vi "Stop Core.vi"(10 "final error code":i32, 11 "Thermocouples in":refnum<class "Thermocouples.lvclass">=refnum) -> (3 "Thermocouples out":refnum<class "Thermocouples.lvclass">)   [LabVIEW 2015]
doc: "(<B>Filename</B>: Actor Framework.lvlib:Actor.lvclass:Stop Core.vi)\n\nDefines what the actor does before it stops. Use the <B>final error code</B> input to determine whether the actor shut down in response to an error.\n\nBy default, this method does nothing. A descendant class may override it to define behavior, such as shutting down any processes the actor initiated in its override of the Actor Core method."
uses:
  Thermocouples.lvclass
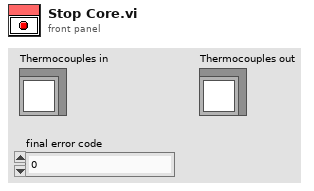
[diagram p1: front panel]
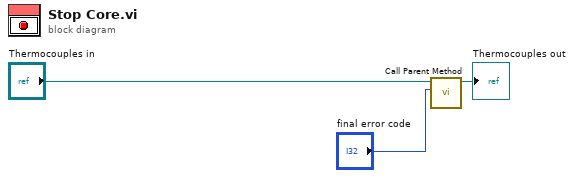
[diagram p0: block diagram]
diagram:
  n1 = call-parent "Call Parent Method"("final error code"="final error code", "AMS Gas Actor in"="Thermocouples in") -> ("AMS Gas Actor out"=→"Thermocouples out":refnum<class "Thermocouples.lvclass">)  [unwired: 9 in]
